vi "Execute Highlight Bookmark.vi"(8 "Error In":errorcluster, 10 "Data":variant, 11 "State In":T1) -> (0 "Error Out":errorcluster, 3 "State Out":T1)   [LabVIEW 2018, in "Bookmark Manager.lvlib"]
uses:
  Bookmark Manager.lvlib
  Controls/State.ctl
  <vilib>/addons/analyzer/_analyzerctrls.llb/VIAnCtl Analysis App Info.ctl
  Controls/Bookmark.ctl
  Controls/VI Identifier.ctl
  Controls/Bookmarks Groups.ctl
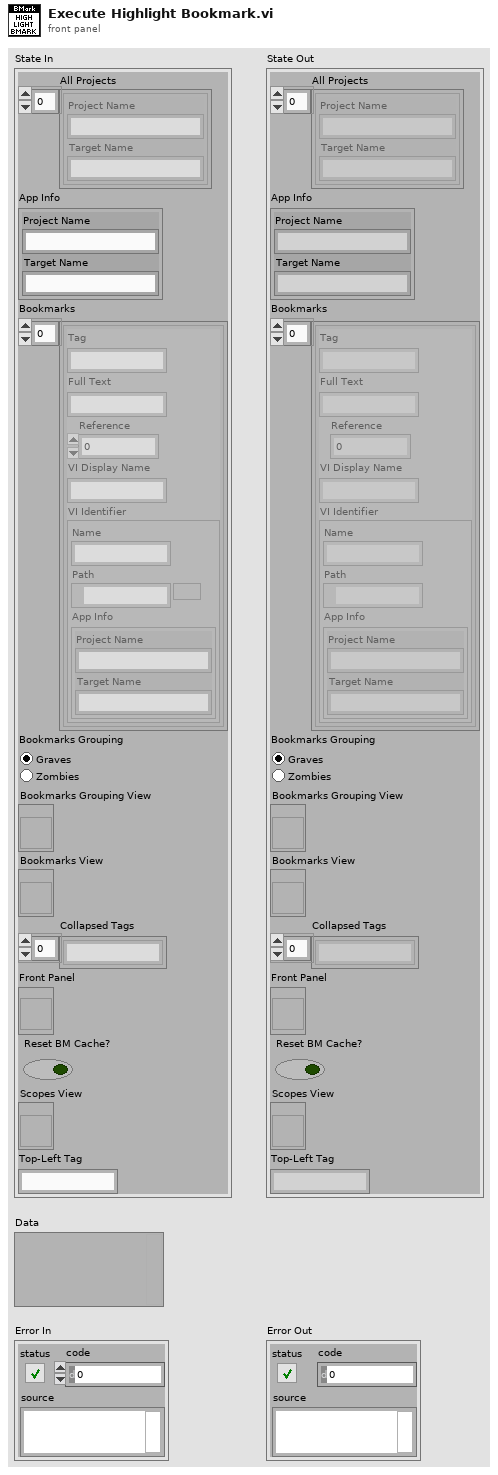
[diagram p1: front panel]
types:
  T1 = typedef "Bookmark Manager.lvlib/State.ctl" = cluster{"All Projects":T2[], "App Info":T2, "Bookmarks":T3[], "Bookmarks Grouping":T5, "Bookmarks Grouping View":refnum<vi>, "Bookmarks View":refnum<vi>, "Collapsed Tags":string[], "Front Panel":refnum<vi>, "Reset BM Cache?":bool, "Scopes View":refnum<vi>, "Top-Left Tag":string}
  T2 = typedef "VIAnCtl Analysis App Info.ctl" = cluster{"Project Name":string, "Target Name":string}
  T3 = typedef "Bookmark Manager.lvlib/Bookmark.ctl" = cluster{"Tag":string, "Full Text":string, "Reference":i32, "VI Display Name":string, "VI Identifier":T4}
  T4 = typedef "Bookmark Manager.lvlib/VI Identifier.ctl" = cluster{"Name":string, "Path":path, "App Info":T2}
  T5 = typedef "Bookmark Manager.lvlib/Bookmarks Groups.ctl" = enum32{"Graves", "Zombies"}
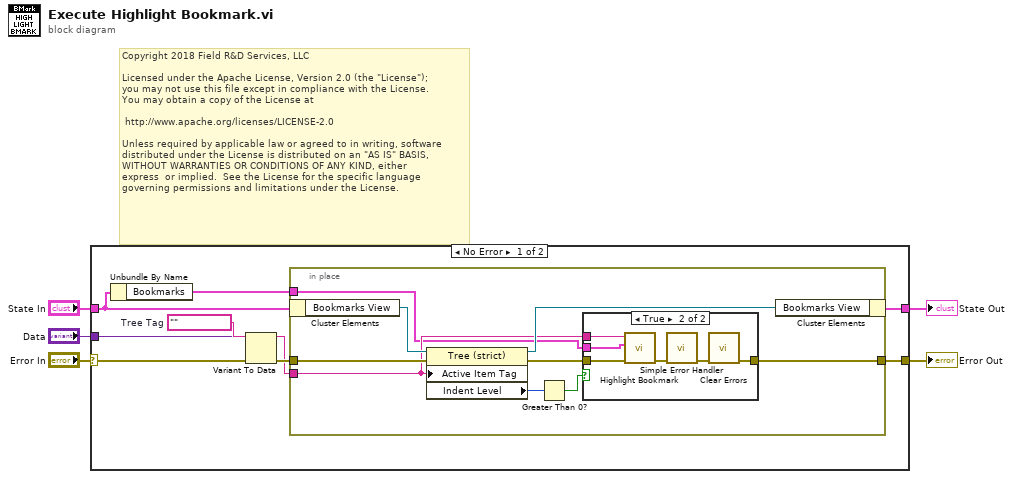
[diagram p0: block diagram]
diagram:
  # "Copyright 2018 Field R&D Services, LLC\n\nLicensed under the Apache License, Version 2.0 (the \"License\");\nyou may not use this file except in compliance with the License.\nYou may obtain a copy of the License at\n\n\thttp://www.apache.org/licenses/LICENSE-2.0\n\nUnless required by applicable law or agreed to in writing, software\ndistributed under the License is distributed on an \"AS IS\" BASIS,\nWITHOUT WARRANTIES OR CONDITIONS OF ANY KIND, either \nexpress  or implied.  See the License for the specific language \ngoverning permissions and limitations under the License."
  n1 = case shown="No Error" "Error In" {
    selector: "Error In" -> [w6 w31]
    tunnel: [w14 w31] -> w5
    tunnel: "Data" -> [w9 _]
    tunnel: "State In" -> [w8 w32]
    tunnel: [w7 w32] -> w2
    frame No Error {
      w10 = ""  # Tree Tag
      n2 = Unbundle By Name(w8) -> ("Bookmarks"=w13:T3[])
      n3 = Variant To Data(error in=w6, type=w10, Variant=w9) -> (data=w11:string, error out=w12:errorcluster)
      n4 = in-place {
        in-place-border: w11 -> [w17]
        in-place-border: w12 -> [w21]
        in-place-border: w13 -> [w16]
        in-place-border: [w15] -> w14
        n5 = in-place-cluster #1(w8) -> ("Bookmarks View"=w23:refnum<vi>)
        n6 = property class="Tree (strict)"(reference=w23, error in=w21, "Active Item Tag"=w17) -> (reference out=w22:refnum<vi>, error out=w18:errorcluster, "Indent Level"=w20:i32)
        n7 = Greater Than 0?(x=w20) -> (x > 0?=w19:bool)
        n8 = case shown="True" w19 {
          tunnel: w18 -> [w24 w28]
          tunnel: w17 -> [_ w30]
          tunnel: w16 -> [_ w29]
          tunnel: [w24 w25] -> w15
          frame False {
          }
          frame True {
            n9 = call "Highlight Bookmark.vi"("Error In"=w28, "Bookmarks"=w29, "Tag"=w30) -> ("Error Out"=w27:errorcluster)  [unwired: 8 in]
            n10 = call <vilib>:"Simple Error Handler.vi"("error in (no error)"=w27) -> ("error out"=w26:errorcluster)  [unwired: 4 in, 4 out]
            n11 = call <vilib>:"Clear Errors.vi"("error in (no error)"=w26) -> ("error out"=w25:errorcluster)  [unwired: 5 in, 1 out]
          }
        }
        n12 = in-place-cluster #1("Bookmarks View"=w22) -> (w7:T1)
      }
    }
    frame Error {
    }
  }
  "Error Out" <- w5
  "State Out" <- w2
